vi "TestAdd.vi"   [LabVIEW 2016, in "SimpleCalculatorTests.lvlib"]
uses:
  SimpleCalculatorTests.lvlib
  main/apis/Stimulus/ValueSignal/ValueSignalByPathString.vi
  main/apis/Stimulus/KeyBoardSimulation/ValueSignalLatchBooleanString.vi
  main/apis/Assert/AssertControlValue/AlmostEqual.vi
  main/Drona.lvlib
  main/apis/Stimulus/ValueSignal/ValueSignal.lvlib
  <vilib>/addons/_JKI Toolkits/Caraya/classes/Test/Test.lvclass
  main/apis/Stimulus/KeyBoardSimulation/KeyboardSimulation.lvlib
  main/apis/Assert/AssertControlValue/AssertControlValue.lvlib
panel:
  # "Drona Test Add"
types:
  T1 = cluster{"Input 1":dbl, "Input 2":dbl, "Output":dbl}[]
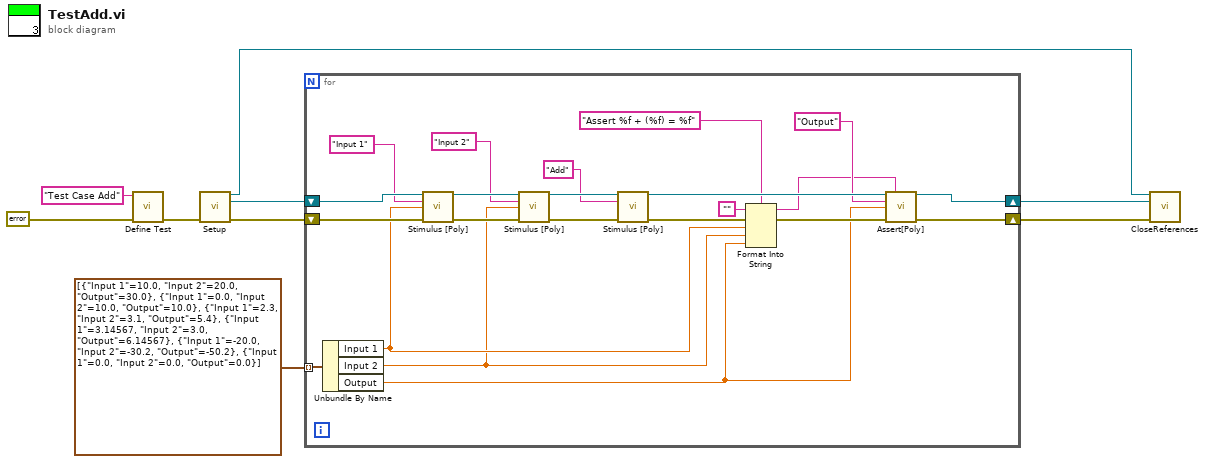
[diagram p0: block diagram]
diagram:
  n1 = call <vilib>:"Define Test.vi"("error in (no error)"=errorcluster {"status"=FALSE, "code"=0, "source"=""} ("error in"), "Label (VI Title)"="Test Case Add") -> ("error out"=w3:errorcluster)  [unwired: 9 in]
  n2 = call "Setup.vi"("error in"=w3) -> ("Application Ref"=w7:refnum<vi>, "VI Reference Out"=w9:refnum<vi>, "error out"=w8:errorcluster)  [unwired: 12 in]
  n3 = for {
    shift-right: [w19] -> w4
    shift-left: w9 -> [w31]
    shift-right: [w21] -> w5
    shift-left: w8 -> [w30]
    tunnel: T1 [{"Input 1"=10.0, "Input 2"=20.0, "Output"=30.0}, {"Input 1"=0.0, "Input 2"=10.0, "Output"=10.0}, {"Input 1"=2.3, "Input 2"=3.1, "Output"=5.4}, {"Input 1"=3.14567, "Input 2"=3.0, "Output"=6.14567}, {"Input 1"=-20.0, "Input 2"=-30.2, "Output"=-50.2}, {"Input 1"=0.0, "Input 2"=0.0, "Output"=0.0}] -> [w17] mode=indexing
    n4 = Unbundle By Name(w17) -> ("Input 1"=w14:dbl, "Input 2"=w13:dbl, "Output"=w12:dbl)
    n5 = call-poly "Stimulus [Poly].vi"("VI Reference In"=w31, "Control Path"="Input 1", "Value (Signaling)"=w14, "error in"=w30) -> ("VI Reference Out"=w27:refnum<vi>, "error out"=w28:errorcluster)  [unwired: 10 in]
    n6 = call-poly "Stimulus [Poly].vi"("VI Reference In"=w27, "Control Path"="Input 2", "Value (Signaling)"=w13, "error in"=w28) -> ("VI Reference Out"=w25:refnum<vi>, "error out"=w24:errorcluster)  [unwired: 10 in]
    n7 = call-poly "Stimulus [Poly].vi"("VI Reference In"=w25, "Control Path"="Add", "error in"=w24) -> ("VI Reference Out"=w20:refnum<vi>, "error out"=w22:errorcluster)  [unwired: 11 in]
    n8 = Format Into String(format string="Assert %f + (%f) = %f", initial string="", error in=w22, w14, w13, w12) -> (resulting string=w11:string, error out=w16:errorcluster)
    n9 = call-poly "Assert[Poly].vi"("VI Reference In"=w20, "Label"=w11, "Control Path"="Output", "Control Value"=w12, "Error In"=w16) -> ("VI Reference Out"=w19:refnum<vi>, "Error Out"=w21:errorcluster)  [unwired: 9 in]
  }
  n10 = call "CloseReferences.vi"("Application Ref"=w7, "VI Reference Out"=w4, "error in"=w5) -> ()  [unwired: 12 in, 1 out]
